vi "force_control_loop.vi"(0 "Force In":dbl[](array[numeric]), 5 "Goal Position IN":dbl[][](array[numeric]), 7 "Force Stimulus":dbl[](array[numeric])) -> (6 "Force Position Out":dbl[](array[numeric]), 15 "Last Error":dbl[](array[numeric]))   [LabVIEW 2013]
uses:
  <vilib>/Analysis/NI_AALBase.lvlib
  <vilib>/Analysis/baseanly.llb/Real A x B.vi
  <vilib>/Analysis/Matrix/NI_Matrix.lvlib
  <vilib>/Analysis/Matrix/Numeric/Conversions/Matrix To Array - RM.vi
  force_control_globals.vi
  <vilib>/Analysis/Matrix/Datatypes/RealMatrix.ctl
panel:
  out "Goal Position HOLD":dbl[][](array[numeric])
  out "Last dForce":dbl[](array[numeric])
  out "Inject Stimulus":bool
  out "Last Force":dbl[](array[numeric])
  in  "Accel Transform":T1
  out "Last Ki":dbl[](array[numeric])
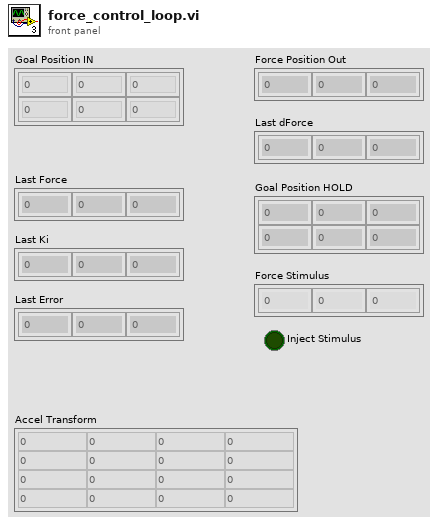
[diagram p1: front panel]
types:
  T1 = typedef "NI_Matrix.lvlib/RealMatrix.ctl" = dbl[][]
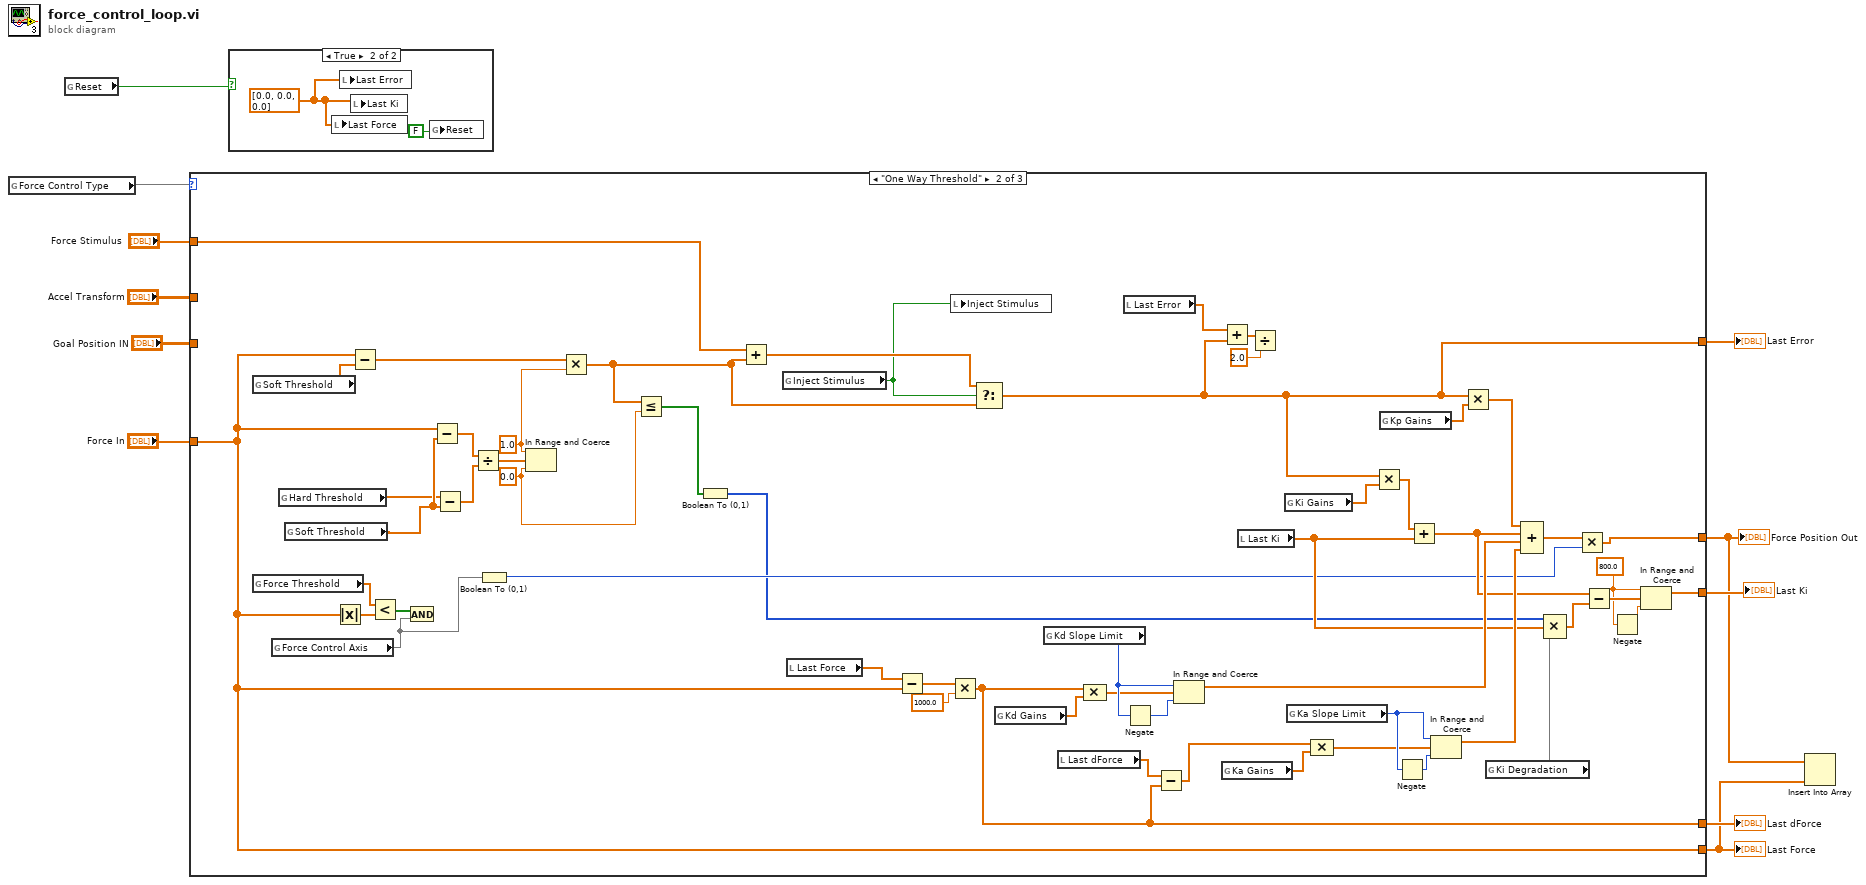
[diagram p0: block diagram]
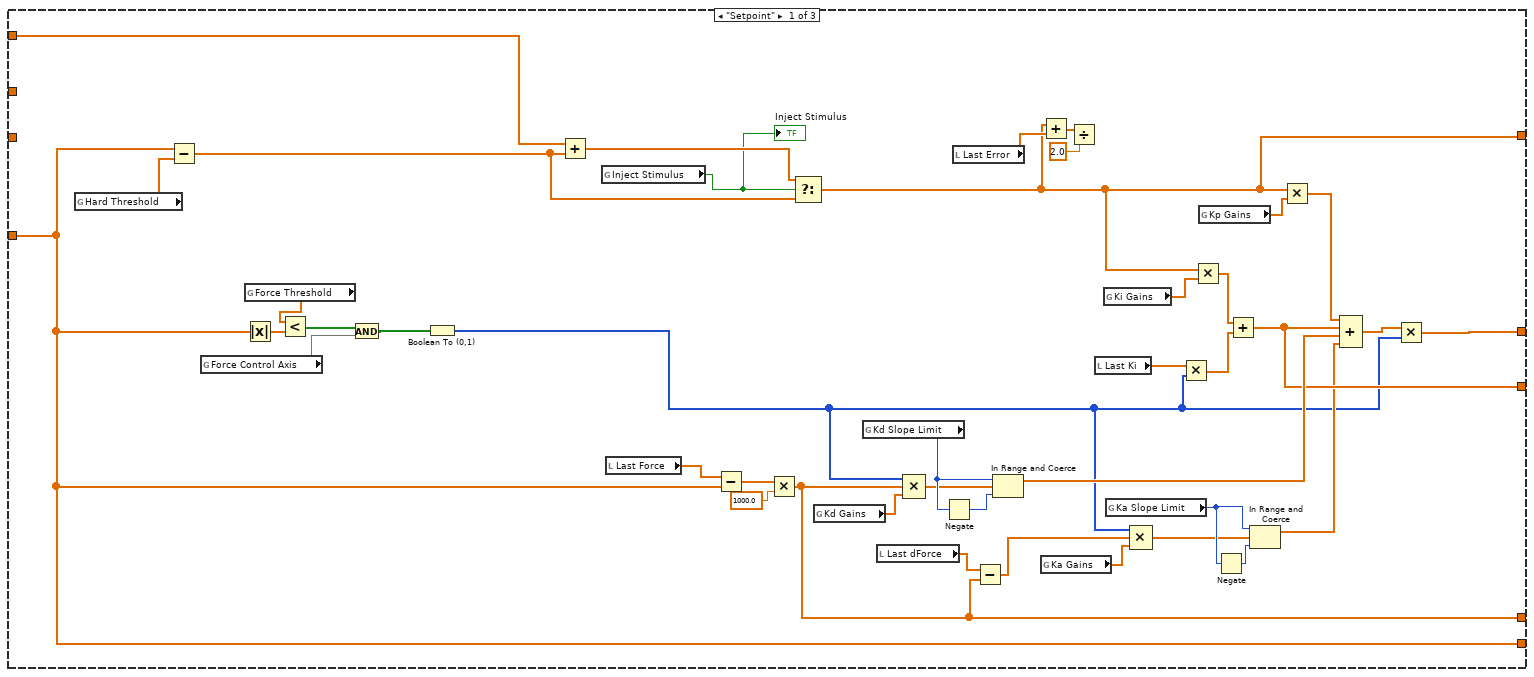
[diagram p3: hidden frame]
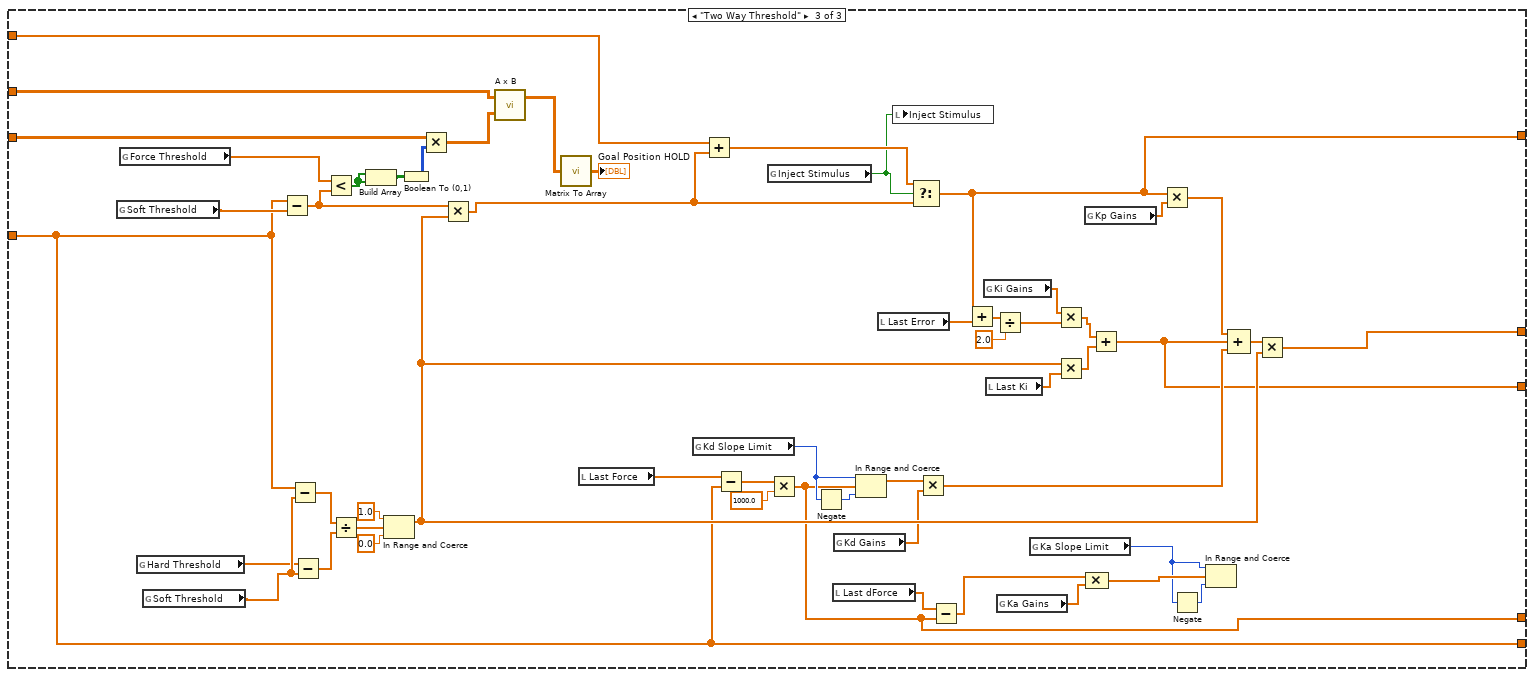
[diagram p4: hidden frame]
diagram:
  n1 = global read "force_control_globals.vi" "Force Control Type"() -> (w10)
  n2 = global read "force_control_globals.vi" "Reset"() -> (w5:bool)
  n3 = case shown="\"One Way Threshold\"" w10 {
    tunnel: "Force In" -> [w34 w75 w111]
    tunnel: [w28 w56 w108] -> w4
    tunnel: [w27 w70 w146] -> w7
    tunnel: [w30 w58 w144] -> w2
    tunnel: "Accel Transform" -> [_ _ w131]
    tunnel: "Force Stimulus" -> [w41 w97 w119]
    tunnel: [w34 w75 w111] -> w1
    tunnel: "Goal Position IN" -> [_ _ w117]
    tunnel: [w22 w86 w110] -> w6
    frame "Setpoint" {
      n4 = global read "force_control_globals.vi" "Hard Threshold"() -> (w39:sgl[])
      n5 = Subtract(x=w34, y=w39) -> (x-y=w36:dbl[])
      n6 = global read "force_control_globals.vi" "Force Control Axis"() -> (w13)
      n7 = global read "force_control_globals.vi" "Force Threshold"() -> (w16:sgl[])
      n8 = Absolute Value(x=w34) -> (abs(x)=w52:dbl[])
      n9 = Less?(x=w16, y=w52) -> (x < y?=w14:bool[])
      n10 = And(x=w14, y=w13) -> (x .and. y?=w15:bool[])
      n11 = Boolean To (0,1)(Boolean=w15) -> (0, 1=w12:i16[])
      n12 = Add(x=w41, y=w36) -> (x+y=w51:dbl[])
      n13 = global read "force_control_globals.vi" "Inject Stimulus"() -> (w37:bool)
      "Inject Stimulus" <- w37
      n14 = local read "Last Force"() -> (w47:dbl[])
      n15 = Subtract(x=w47, y=w34) -> (x-y=w49:dbl[])
      n16 = Multiply(x=w49, y=1000.0) -> (x*y=w22:dbl[])
      n17 = Select(t=w51, s=w37, f=w36) -> (s? t:f=w27:dbl[])
      n18 = global read "force_control_globals.vi" "Kd Gains"() -> (w38:sgl[])
      n19 = global read "force_control_globals.vi" "Kd Slope Limit"() -> (w33:i32)
      n20 = local read "Last dForce"() -> (w23:dbl[])
      n21 = Compound Arithmetic op=MULTIPLY(w12, w22, w38) -> (w32:dbl[])
      n22 = Negate(x=w33) -> (-x=w46:i32)
      n23 = local read "Last Error"() -> (w43:dbl[])
      n24 = Subtract(x=w23, y=w22) -> (x-y=w21:dbl[])
      n25 = In Range and Coerce(upper limit=w33, x=w32, lower limit=w46) -> (coerced(x)=w31:dbl[])  [unwired: 1 out]
      n26 = Add(x=w27, y=w43) -> (x+y=w44:dbl[])
      n27 = global read "force_control_globals.vi" "Ka Gains"() -> (w24:sgl[])
      n28 = Divide(x=w44, y=2.0) -> ()  [unwired: 1 out]
      n29 = local read "Last Ki"() -> (w25:dbl[])
      n30 = global read "force_control_globals.vi" "Ki Gains"() -> (w35:sgl[])
      n31 = global read "force_control_globals.vi" "Ka Slope Limit"() -> (w19:i32)
      n32 = Compound Arithmetic op=MULTIPLY(w12, w21, w24) -> (w18:dbl[])
      n33 = Multiply(x=w25, y=w12) -> (x*y=w26:dbl[])
      n34 = Multiply(x=w27, y=w35) -> (x*y=w42:dbl[])
      n35 = global read "force_control_globals.vi" "Kp Gains"() -> (w40:sgl[])
      n36 = Negate(x=w19) -> (-x=w20:i32)
      n37 = Add(x=w42, y=w26) -> (x+y=w28:dbl[])
      n38 = In Range and Coerce(upper limit=w19, x=w18, lower limit=w20) -> (coerced(x)=w17:dbl[])  [unwired: 1 out]
      n39 = Multiply(x=w27, y=w40) -> (x*y=w50:dbl[])
      n40 = Compound Arithmetic op=ADD(w50, w28, w31, w17) -> (w29:dbl[])
      n41 = Multiply(x=w29, y=w12) -> (x*y=w30:dbl[])
    }
    frame "One Way Threshold" {
      w53 = 800.0
      w71 = 1.0 ("upper limit")
      w61 = 0.0 ("lower limit")
      n42 = global read "force_control_globals.vi" "Soft Threshold"() -> (w95:sgl[])
      n43 = global read "force_control_globals.vi" "Force Threshold"() -> (w80:sgl[])
      n44 = global read "force_control_globals.vi" "Force Control Axis"() -> (w62)
      n45 = global read "force_control_globals.vi" "Hard Threshold"() -> (w77:sgl[])
      n46 = global read "force_control_globals.vi" "Soft Threshold"() -> (w78:sgl[])
      n47 = Absolute Value(x=w75) -> (abs(x)=w107:dbl[])
      n48 = Subtract(x=w75, y=w95) -> (x-y=w74:dbl[])
      n49 = Less?(x=w80, y=w107) -> (x < y?=w69:bool[])
      n50 = And(x=w69, y=w62) -> ()  [unwired: 1 out]
      n51 = Subtract(x=w75, y=w78) -> (x-y=w76:dbl[])
      n52 = Subtract(x=w77, y=w78) -> (x-y=w63:sgl[])
      n53 = Divide(x=w76, y=w63) -> (x/y=w79:dbl[])
      n54 = Boolean To (0,1)(Boolean=w62) -> (0, 1=w60:i16)
      n55 = In Range and Coerce(upper limit=w71, x=w79, lower limit=w61) -> ()  [unwired: 2 out]
      n56 = Multiply(x=w74, y=w71) -> (x*y=w65:dbl[])
      n57 = Less Or Equal?(x=w65, y=w61) -> (x <= y?=w64:bool[])
      n58 = Boolean To (0,1)(Boolean=w64) -> (0, 1=w59:i16[])
      n59 = Add(x=w97, y=w65) -> (x+y=w106:dbl[])
      n60 = global read "force_control_globals.vi" "Inject Stimulus"() -> (w73:bool)
      n61 = local read "Last Force"() -> (w102:dbl[])
      n62 = Subtract(x=w102, y=w75) -> (x-y=w104:dbl[])
      n63 = Multiply(x=w104, y=1000.0) -> (x*y=w86:dbl[])
      n64 = local write "Inject Stimulus"(w73) -> ()
      n65 = Select(t=w106, s=w73, f=w65) -> (s? t:f=w70:dbl[])
      n66 = global read "force_control_globals.vi" "Kd Gains"() -> (w94:sgl[])
      n67 = global read "force_control_globals.vi" "Kd Slope Limit"() -> (w92:i32)
      n68 = local read "Last dForce"() -> (w87:dbl[])
      n69 = Compound Arithmetic op=MULTIPLY(w86, w94) -> (w91:dbl[])
      n70 = local read "Last Error"() -> (w72:dbl[])
      n71 = Negate(x=w92) -> (-x=w101:i32)
      n72 = Subtract(x=w87, y=w86) -> (x-y=w85:dbl[])
      n73 = In Range and Coerce(upper limit=w92, x=w91, lower limit=w101) -> (coerced(x)=w90:dbl[])  [unwired: 1 out]
      n74 = Add(x=w72, y=w70) -> (x+y=w99:dbl[])
      n75 = global read "force_control_globals.vi" "Ka Gains"() -> (w88:sgl[])
      n76 = local read "Last Ki"() -> (w67:dbl[])
      n77 = Divide(x=w99, y=2.0) -> ()  [unwired: 1 out]
      n78 = global read "force_control_globals.vi" "Ki Gains"() -> (w93:sgl[])
      n79 = global read "force_control_globals.vi" "Ka Slope Limit"() -> (w83:i32)
      n80 = Compound Arithmetic op=MULTIPLY(w85, w88) -> (w82:dbl[])
      n81 = Multiply(x=w70, y=w93) -> (x*y=w98:dbl[])
      n82 = global read "force_control_globals.vi" "Kp Gains"() -> (w96:sgl[])
      n83 = Negate(x=w83) -> (-x=w84:i32)
      n84 = Add(x=w98, y=w67) -> (x+y=w68:dbl[])
      n85 = In Range and Coerce(upper limit=w83, x=w82, lower limit=w84) -> (coerced(x)=w81:dbl[])  [unwired: 1 out]
      n86 = Multiply(x=w70, y=w96) -> (x*y=w105:dbl[])
      n87 = global read "force_control_globals.vi" "Ki Degradation"() -> (w57)
      n88 = Compound Arithmetic op=ADD(w105, w68, w90, w81) -> (w89:dbl[])
      n89 = Compound Arithmetic op=MULTIPLY(w59, w67, w57) -> (w66:dbl[])
      n90 = Multiply(x=w89, y=w60) -> (x*y=w58:dbl[])
      n91 = Subtract(x=w68, y=w66) -> (x-y=w55:dbl[])
      n92 = Negate(x=w53) -> (-x=w54:dbl)
      n93 = In Range and Coerce(upper limit=w53, x=w55, lower limit=w54) -> (coerced(x)=w56:dbl[])  [unwired: 1 out]
    }
    frame "Two Way Threshold" {
      n94 = global read "force_control_globals.vi" "Soft Threshold"() -> (w121:sgl[])
      n95 = global read "force_control_globals.vi" "Force Threshold"() -> (w120:sgl[])
      n96 = global read "force_control_globals.vi" "Hard Threshold"() -> (w122:sgl[])
      n97 = global read "force_control_globals.vi" "Soft Threshold"() -> (w123:sgl[])
      n98 = Subtract(x=w111, y=w121) -> (x-y=w135:dbl[])
      n99 = Subtract(x=w111, y=w123) -> (x-y=w140:dbl[])
      n100 = Subtract(x=w122, y=w123) -> (x-y=w139:sgl[])
      n101 = Less?(x=w120, y=w135) -> (x < y?=w134:bool[])
      n102 = Divide(x=w140, y=w139) -> (x/y=w138:dbl[])
      n103 = Build Array(w134, w134) -> (w132:bool[][])
      n104 = In Range and Coerce(upper limit=1.0, x=w138, lower limit=0.0) -> (coerced(x)=w136:dbl[])  [unwired: 1 out]
      n105 = Boolean To (0,1)(Boolean=w132) -> (0, 1=w133:i16[][])
      n106 = Multiply(x=w117, y=w133) -> (x*y=w130:dbl[][])
      n107 = Multiply(x=w135, y=w136) -> (x*y=w137:dbl[])
      n108 = call-poly <vilib>:"A x B.vi"("B"=w130, "A"=w131) -> ("A x B"=w128:T1)  [unwired: 1 out]
      n109 = call-poly <vilib>:"Matrix To Array.vi"("Real Matrix"=w128) -> ("Real 2D Array"=→"Goal Position HOLD":dbl[][])
      n110 = local read "Last Force"() -> (w155:dbl[])
      n111 = global read "force_control_globals.vi" "Kd Slope Limit"() -> (w124:i32)
      n112 = Add(x=w119, y=w137) -> (x+y=w160:dbl[])
      n113 = Subtract(x=w155, y=w111) -> (x-y=w157:dbl[])
      n114 = global read "force_control_globals.vi" "Inject Stimulus"() -> (w118:bool)
      n115 = Multiply(x=w157, y=1000.0) -> (x*y=w110:dbl[])
      n116 = Negate(x=w124) -> (-x=w154:i32)
      n117 = local read "Last dForce"() -> (w115:dbl[])
      n118 = global read "force_control_globals.vi" "Kd Gains"() -> (w125:sgl[])
      n119 = In Range and Coerce(upper limit=w124, x=w110, lower limit=w154) -> (coerced(x)=w153:dbl[])  [unwired: 1 out]
      n120 = local read "Last Error"() -> (w148:dbl[])
      n121 = local write "Inject Stimulus"(w118) -> ()
      n122 = Select(t=w160, s=w118, f=w137) -> (s? t:f=w146:dbl[])
      n123 = Multiply(x=w153, y=w125) -> (x*y=w158:dbl[])
      n124 = Subtract(x=w115, y=w110) -> (x-y=w114:dbl[])
      n125 = Add(x=w146, y=w148) -> (x+y=w149:dbl[])
      n126 = global read "force_control_globals.vi" "Ki Gains"() -> (w126:sgl[])
      n127 = local read "Last Ki"() -> (w151:dbl[])
      n128 = Divide(x=w149, y=2.0) -> (x/y=w147:dbl[])
      n129 = global read "force_control_globals.vi" "Ka Gains"() -> (w116:sgl[])
      n130 = global read "force_control_globals.vi" "Ka Slope Limit"() -> (w109:i32)
      n131 = Multiply(x=w126, y=w147) -> (x*y=w143:dbl[])
      n132 = Multiply(x=w136, y=w151) -> (x*y=w152:dbl[])
      n133 = global read "force_control_globals.vi" "Kp Gains"() -> (w127:sgl[])
      n134 = Compound Arithmetic op=MULTIPLY(w114, w116) -> (w112:dbl[])
      n135 = Add(x=w143, y=w152) -> (x+y=w108:dbl[])
      n136 = Multiply(x=w146, y=w127) -> (x*y=w159:dbl[])
      n137 = Negate(x=w109) -> (-x=w113:i32)
      n138 = In Range and Coerce(upper limit=w109, x=w112, lower limit=w113) -> ()  [unwired: 2 out]
      n139 = Compound Arithmetic op=ADD(w159, w108, w158) -> (w145:dbl[])
      n140 = Multiply(x=w145, y=w136) -> (x*y=w144:dbl[])
    }
  }
  "Last Error" <- w7
  "Last Ki" <- w4
  "Force Position Out" <- w2
  "Last Force" <- w1
  "Last dForce" <- w6
  n141 = case shown="True" w5 {
    frame False {
    }
    frame True {
      w162 = dbl[] [0.0, 0.0, 0.0]
      n142 = local write "Last Force"(w162) -> ()
      n143 = local write "Last Error"(w162) -> ()
      n144 = local write "Last Ki"(w162) -> ()
      n145 = global write "force_control_globals.vi" "Reset"(FALSE) -> ()
    }
  }
  n146 = Insert Into Array(array=w2, new element=w1) -> ()  [unwired: 1 in, 1 out]
